vi "Handle Error.vi"(8 "error in (no error)":errorcluster, 11 "output_actor_errorneous in":refnum<class "Output Actor Hardware.lvclass">) -> (0 "error out":errorcluster, 2 "stop actor?":bool=TRUE, 3 "output_actor_errorneous out":refnum<class "Output Actor Hardware.lvclass">)   [LabVIEW 2015, in "Output Actor Hardware.lvclass"]
doc: "(<B>Filename</B>: Actor Framework.lvlib:Actor.lvclass:Handle Error.vi)\n\nDefines how the actor handles an error that occurred while processing a message. By default, this method does nothing except stop the actor."
uses:
  Output Actor Hardware.lvclass
  state.ctl
panel:
  in  "state":T1
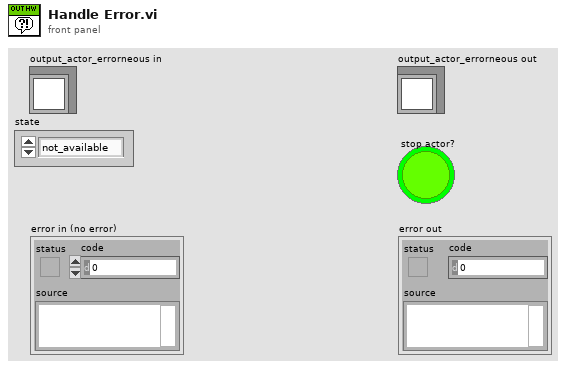
[diagram p1: front panel]
types:
  T1 = typedef "Output Actor Hardware.lvclass/state.ctl" = enum16{"not_available", "not_initialized", "ok"}
  T2 = cluster{"status":bool, "code":bool, "source":bool}
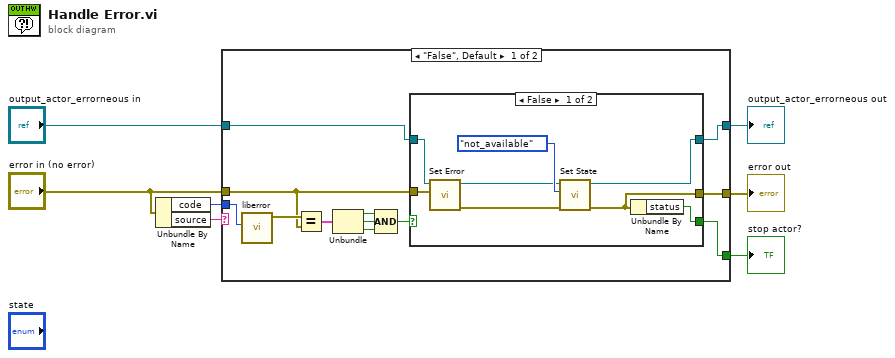
[diagram p0: block diagram]
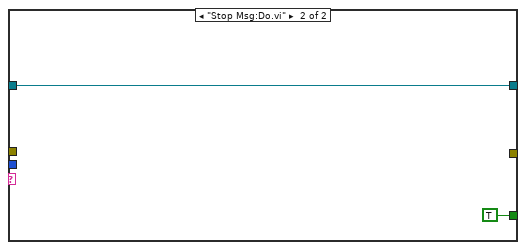
[diagram p3: hidden frame]
diagram:
  n1 = Unbundle By Name("error in (no error)") -> ("code"=w2:i32, "source"=w7:string)
  n2 = case shown="\"False\", Default" w7 {
    tunnel: [w18 TRUE ("x = y?")] -> w6
    tunnel: "output_actor_errorneous in" -> [w19 w31]
    tunnel: [w17 _] -> w4
    tunnel: [w16 w31] -> w3
    tunnel: w2 -> [w15 _]
    tunnel: "error in (no error)" -> [w8 _]
    frame "False", Default {
      n3 = call "liberror.vi"("tvio errors"=w15) -> ("error out"=w14:errorcluster)  [unwired: 10 in]
      n4 = Equal?(x=w14, y=w8) -> (x = y?=w13:T2)
      n5 = Unbundle(w13) -> ("status"=w12:bool, "code"=w11:bool, "source"=w10:bool)
      n6 = Compound Arithmetic op=AND(w12, w11, w10) -> (w9:bool)
      n7 = case shown="False" w9 {
        selector: w9 -> [_ w28]
        tunnel: w19 -> [w23 w30]
        tunnel: [w27 w28] -> w18
        tunnel: [w24 w29] -> w17
        tunnel: [w25 w30] -> w16
        tunnel: w8 -> [w21 w29]
        frame False {
          n8 = call "Set Error.vi"("error"=w21, "Output Actor Hardware in"=w23) -> ("error out"=w20:errorcluster, "Output Actor Hardware out"=w22:refnum<class "Output Actor Hardware.lvclass">)  [unwired: 8 in]
          n9 = call "Set State.vi"("error in (no error)"=w20, "state"=state."not_available", "output_actor_errorneous in"=w22) -> ("error out"=w24:errorcluster, "output_actor_errorneous out"=w25:refnum<class "Output Actor Hardware.lvclass">)  [unwired: 7 in]
          n10 = Unbundle By Name(w24) -> ("status"=w27:bool)
        }
        frame True {
        }
      }
    }
    frame "Stop Msg:Do.vi" {
    }
  }
  "output_actor_errorneous out" <- w3
  "error out" <- w4
  "stop actor?" <- w6
